vi "325-340 Read and Compressor auto control(SubVI) - v1.vi"(11 "Instrument":T3={"325 Resource "="GPIB0::24::INSTR", "Input (0:A) 325"=0, "Heater Output (1:1) 325"=1, "340 Resource"="GPIB0::14::INSTR", "Input (0:A) 340"=1, "Heater Output (1:1) 340"=1, "340 Status"=refnum, "Instrument Type"=enum."PPMS", "quantum design"=refnum, "semaphore 325"=refnum, "TCP master instance"=refnum, "M24C Resource"="GPIB0::24::INSTR", "4G supply"="GPIB0::24::INSTR", "Temp Status 24C"=refnum, "Temp"=refnum, "9T信号"=refnum, "limit"={"Field limit"=0.0, "Field rate limit"=0.0, "Temp limit"=0.0, "Temp low limit"=0.0, "Temp rate limit "=0.0}, "4g supply status"=refnum, "vi路径"="", "in-plane"="", "out-plane"="", "in-plane signal"=FALSE, "out-plane signal"=FALSE, "in plane 信号"=refnum, "pzt volt"=refnum, "Aborting"=refnum, "数据文件"=refnum, "warning"=refnum, "750 visa"="", "750 rotate"="", "335 Status 2"=refnum, "335 Resource "="GPIB0::24::INSTR", "Input (0:A) 335"=0, "Input (0:B) 335"=1, "Heater Output (1:1) 335"=1, "semaphore 340"=refnum, "semaphore 335"=refnum, "325 Status"=refnum} {"Heater Output (1:1) 335" items=["1"=1, "2"=2]; "Input (0:B) 335" items=["A", "B"]; "Input (0:A) 335" items=["A", "B"]; "Heater Output (1:1) 325" items=["1"=1, "2"=2]; "Input (0:A) 325" items=["A", "B"]; "Input (0:A) 340" items=["A", "B", "C", "D"]; "Heater Output (1:1) 340" items=["1", "2"]}) -> (3 "output cluster":T2 {"?" items=["Unknow", "Stable", "Following Warm", "Following Cold", "Unfollowing"]; "?" items=["Unknow", "Stable", "Following Warm", "Following Cold", "Unfollowing"]})   [LabVIEW 2019, in "Get value.lvlib"]
uses:
  Get value.lvlib
  ctl/Instrument.ctl
  <vilib>/NI/Modbus Library/API/Master/Modbus Master.lvclass
  ctl/335 state.ctl
  ctl/Instrument Type.ctl
  C:/Users/whmfc/Desktop/MEASURE/lib/QDInstrument.dll
  lib/QDInstrument.dll
  ctl/limit.ctl
  ctl/9T mag field stauts.ctl
  ctl/warning.ctl
  lib/Lake Shore 325/Lake Shore 325.lvlib
  lib/Lake Shore 340/Lake Shore Cryotronics 340.lvlib
panel:
  out "下拉列表 2":T1=2 items=["Unknow", "Stable", "Following Warm", "Following Cold", "Unfollowing"]
  out "下拉列表":T1=2 items=["Unknow", "Stable", "Following Warm", "Following Cold", "Unfollowing"]
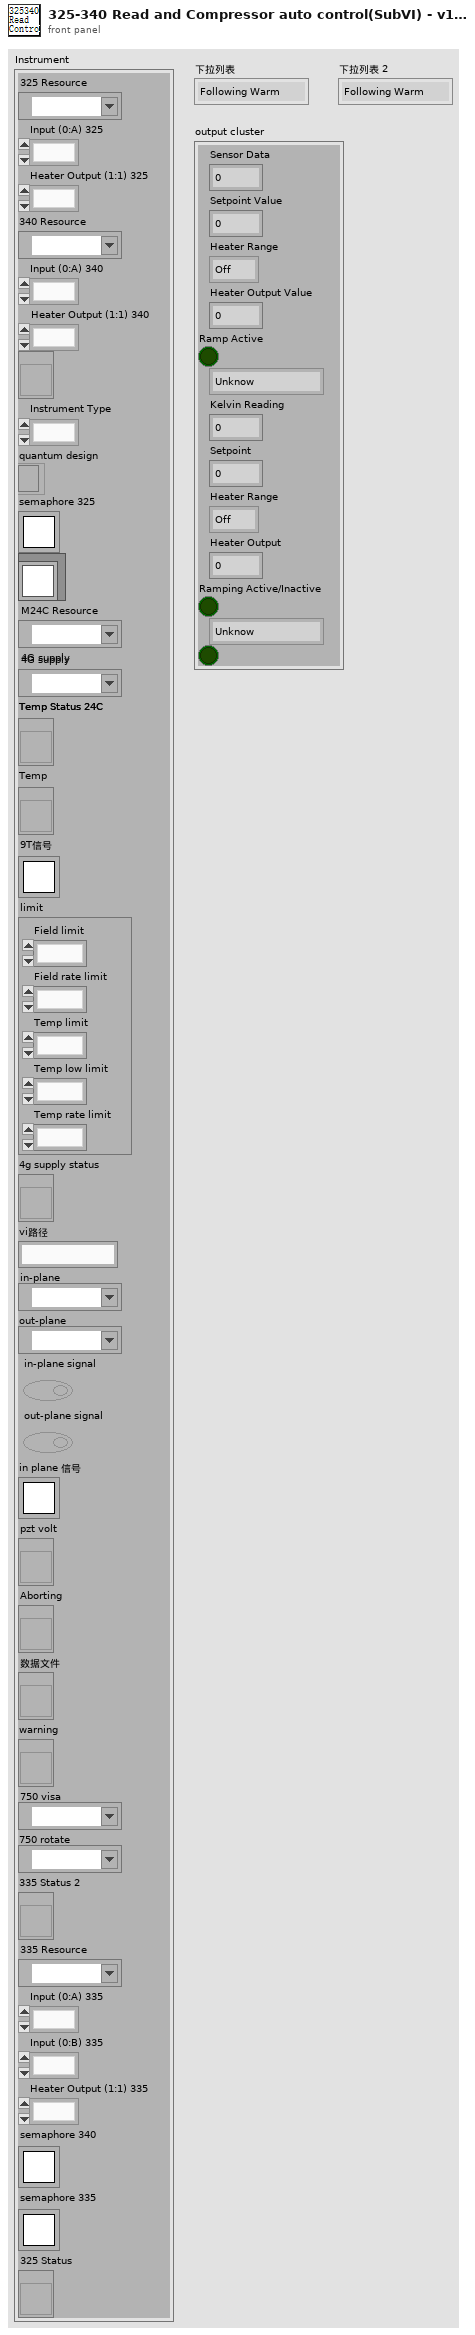
[diagram p1: front panel]
types:
  T1 = typedef "335 state.ctl" = u16
  T2 = cluster{"Sensor Data":dbl, "Setpoint Value":dbl, "Heater Range":enum16{"Off", "Low", "High"}, "Heater Output Value":dbl, "Ramp Active":bool, T1, "Kelvin Reading":dbl, "Setpoint":dbl, "Heater Range":enum16{"Off", "1", "2", "3", "4", "5"}, "Heater Output":dbl, "Ramping Active/Inactive":bool, T1, bool}
  T3 = typedef "Instrument.ctl" = cluster{"325 Resource ":refnum<visa-resource-name>, "Input (0:A) 325":u16, "Heater Output (1:1) 325":u16, "340 Resource":refnum<visa-resource-name>, "Input (0:A) 340":u16, "Heater Output (1:1) 340":u16, "340 Status":refnum<vi>, "Instrument Type":T4, "quantum design":refnum<k24>, "semaphore 325":T5, "TCP master instance":refnum<class "Modbus Master.lvclass">, "M24C Resource":refnum<visa-resource-name>, "4G supply":refnum<visa-resource-name>, "Temp Status 24C":refnum<vi>, "Temp":refnum<vi>, "9T信号":T5, "limit":T6, "4g supply status":refnum<vi>, "vi路径":string, "in-plane":refnum<visa-resource-name>, "out-plane":refnum<visa-resource-name>, "in-plane signal":bool, "out-plane signal":bool, "in plane 信号":T5, "pzt volt":refnum<vi>, "Aborting":refnum<vi>, "数据文件":refnum<vi>, "warning":refnum<vi>, "750 visa":refnum<visa-resource-name>, "750 rotate":refnum<visa-resource-name>, "335 Status 2":refnum<vi>, "335 Resource ":refnum<visa-resource-name>, "Input (0:A) 335":u16, "Input (0:B) 335":u16, "Heater Output (1:1) 335":u16, "semaphore 340":T5, "semaphore 335":T5, "325 Status":refnum<vi>}
  T4 = typedef "Instrument Type.ctl" = enum16{"PPMS", "VersaLab", "DynaCool", "SVSM", "PPMS-Rotate", "Lakeshore335", "lengtou2", "9T mag", "9T cmag rotate", "test"}
  T5 = typedef "Semaphore RefNum" = refnum<k1>
  T6 = typedef "limit.ctl" = cluster{"Field limit":dbl, "Field rate limit":dbl, "Temp limit":dbl, "Temp low limit":dbl, "Temp rate limit ":dbl}
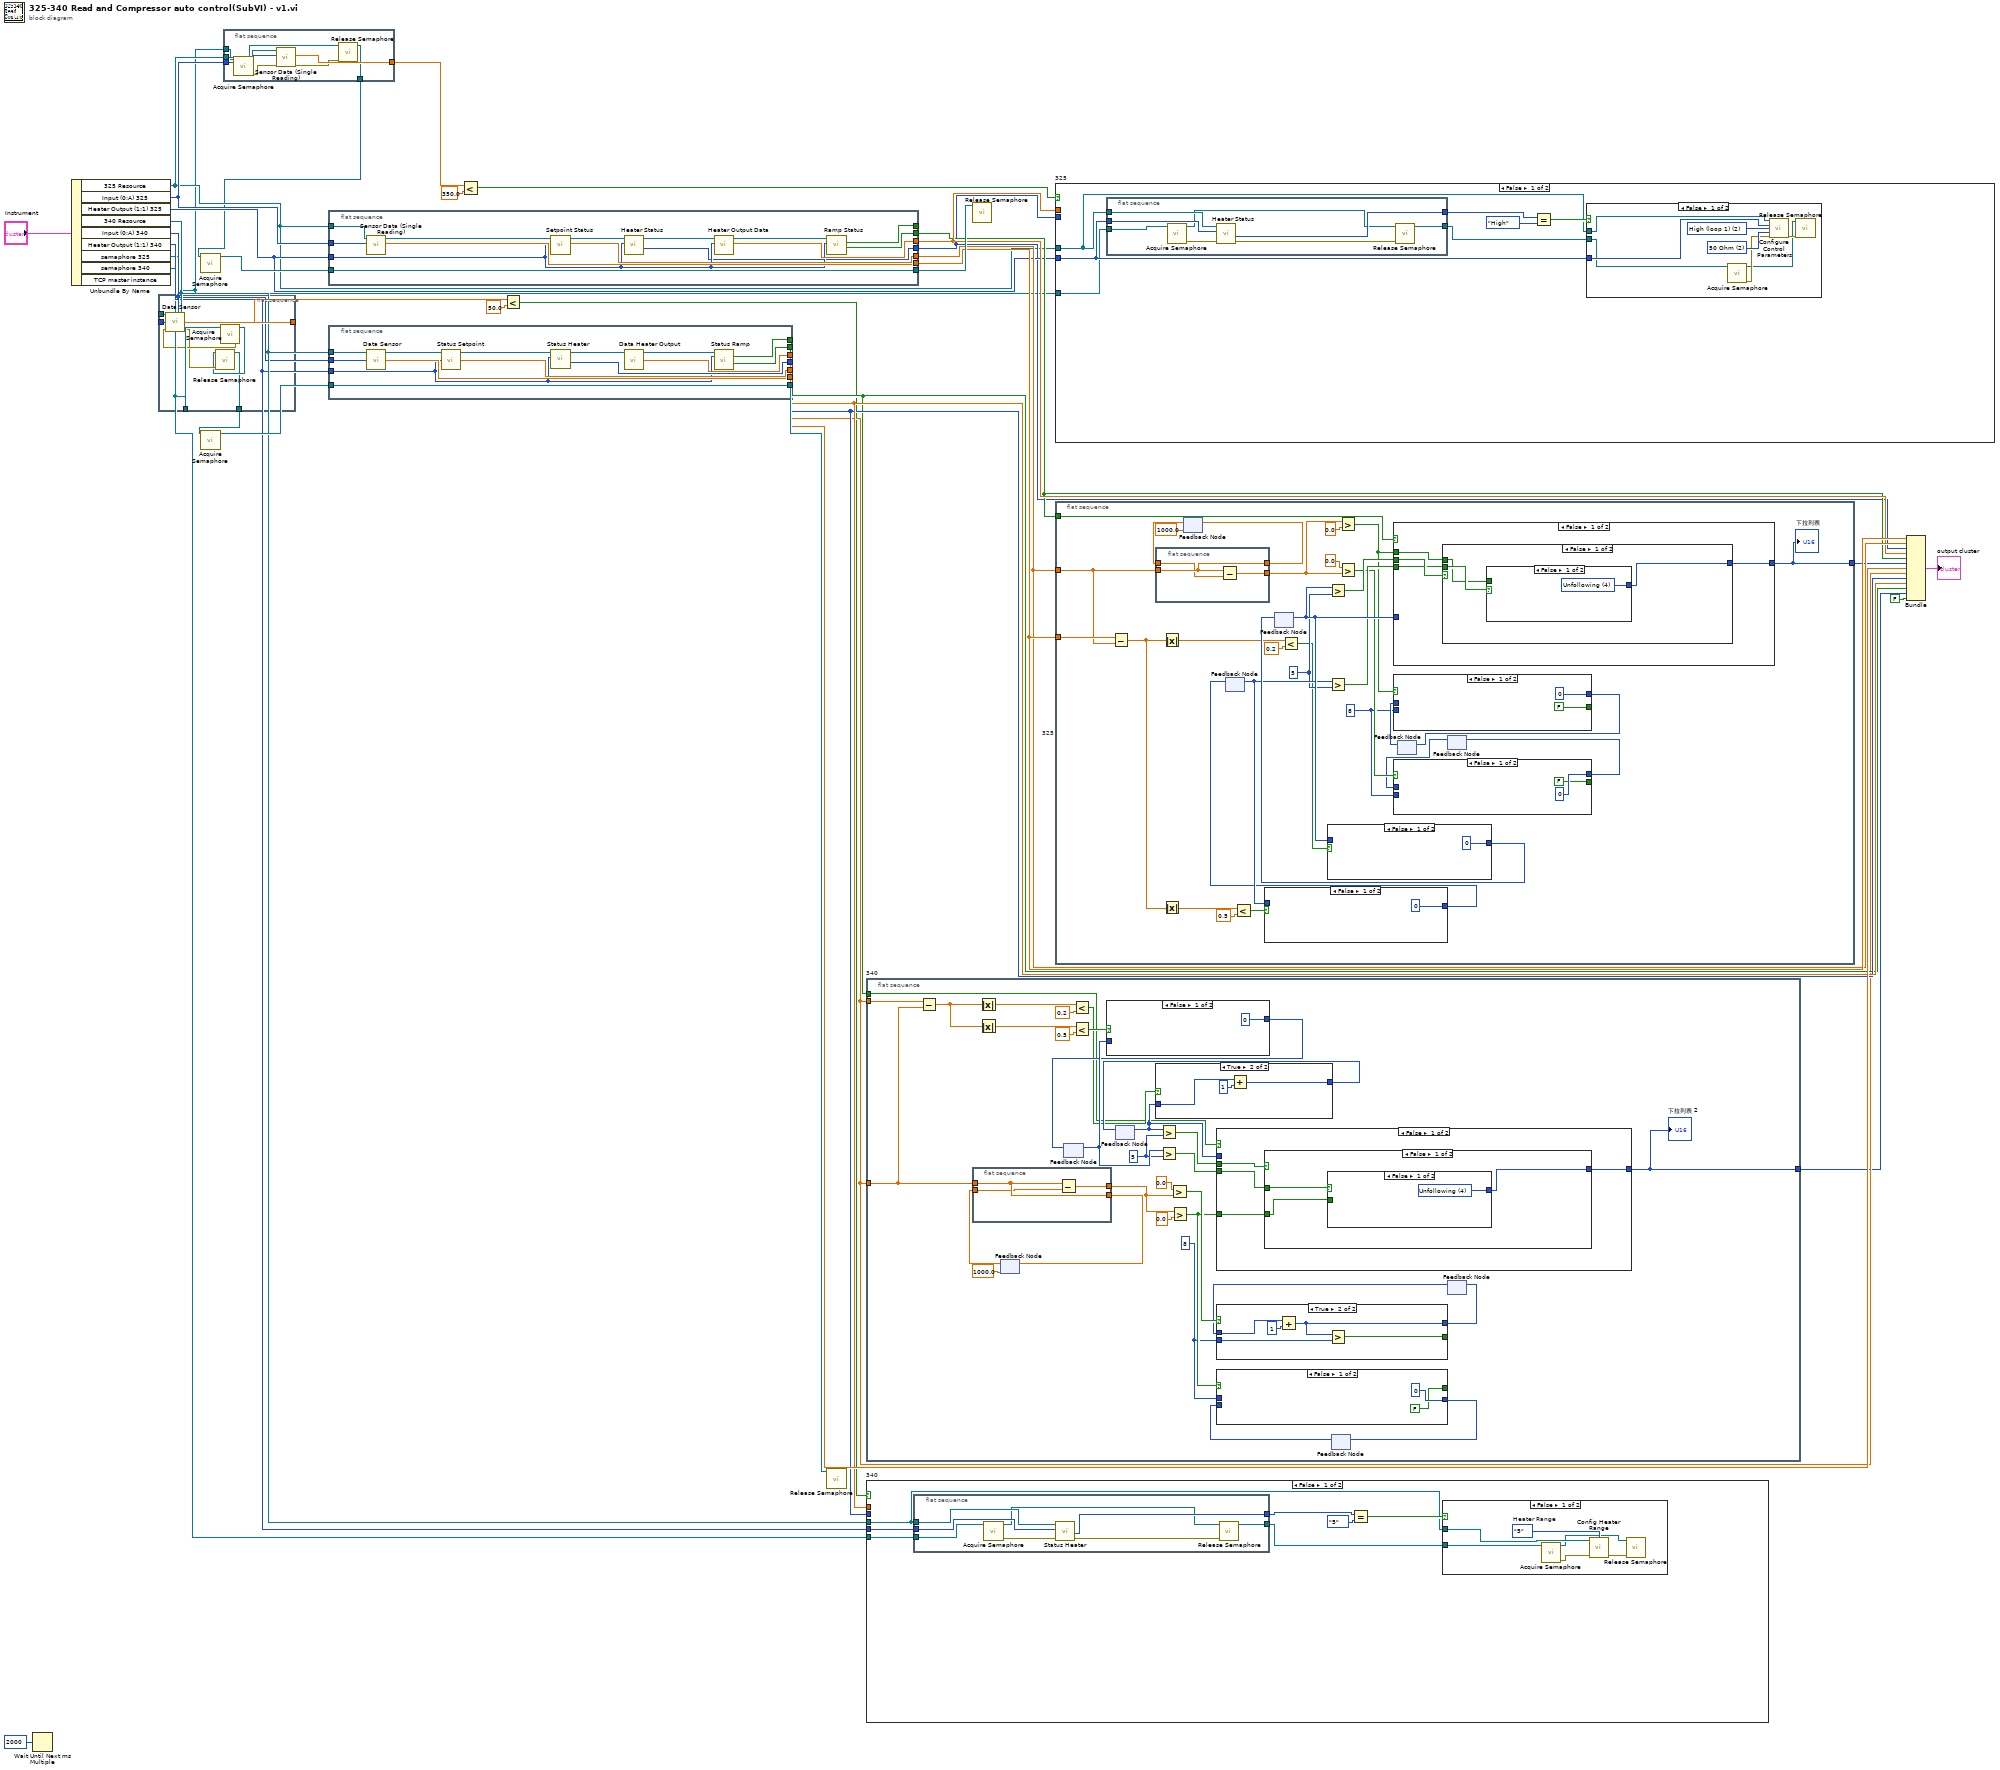
[diagram p0: block diagram]
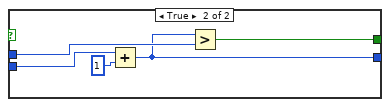
[diagram p2: hidden frame]
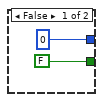
[diagram p3: hidden frame]
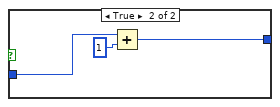
[diagram p4: hidden frame]
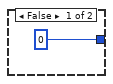
[diagram p5: hidden frame]
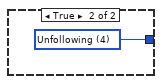
[diagram p6: hidden frame]
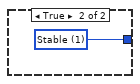
[diagram p7: hidden frame]
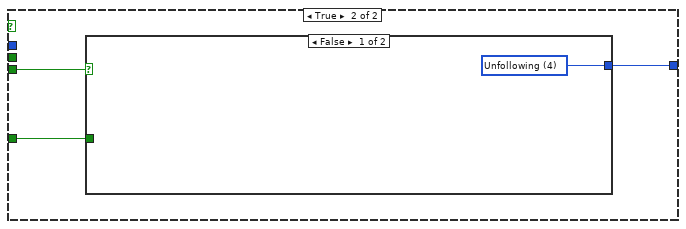
[diagram p8: hidden frame]
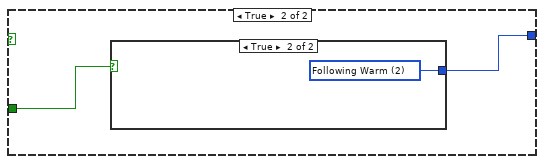
[diagram p9: hidden frame]
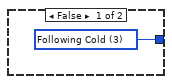
[diagram p10: hidden frame]
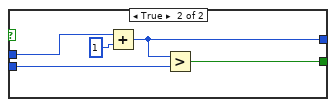
[diagram p11: hidden frame]
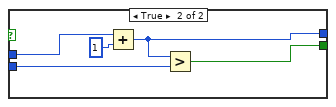
[diagram p12: hidden frame]
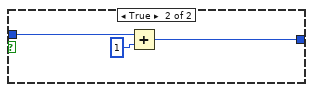
[diagram p13: hidden frame]
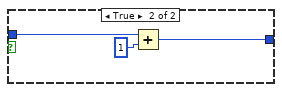
[diagram p14: hidden frame]
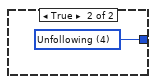
[diagram p15: hidden frame]
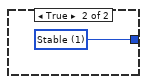
[diagram p16: hidden frame]
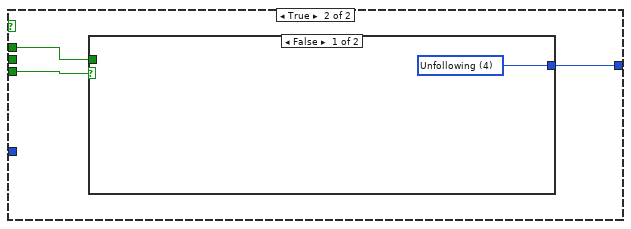
[diagram p17: hidden frame]
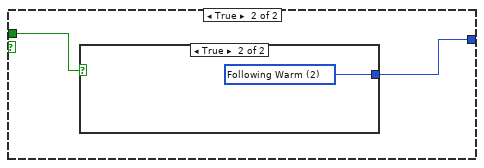
[diagram p18: hidden frame]
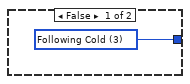
[diagram p19: hidden frame]
diagram:
  n1 = Wait Until Next ms Multiple(millisecond multiple=u32 2000) -> ()  [unwired: 1 out]
  n2 = Unbundle By Name("Instrument") -> ("325 Resource"=w5:refnum<visa-resource-name>, "Input (0:A) 325"=w7:u16, "Heater Output (1:1) 325"=w21:u16, "340 Resource"=w14:refnum<visa-resource-name>, "Input (0:A) 340"=w13:u16, "Heater Output (1:1) 340"=w10:u16, "semaphore 325"=w3:T5, "semaphore 340"=w2:T5)  [unwired: 1 out]
  n3 = flat-sequence {
    tunnel: [w44] -> w15
    tunnel: w14 -> [w43]
    tunnel: w13 -> [w42]
    tunnel: w2 -> [w41]
    tunnel: [w37] -> w1
    frame #0 {
      n4 = call <vilib>:"Acquire Semaphore.vi"("semaphore"=w41) -> ("error out"=w40:errorcluster, "semaphore out"=w38:T5)  [unwired: 4 in, 1 out]
      n5 = call "Data Sensor.vi"("VISA resource name"=w43, "Input (0: A)"=w42, "error in (no error)"=w40) -> ("Kelvin Reading"=w44:dbl, "error out"=w39:errorcluster)  [unwired: 8 in, 3 out]
      n6 = call <vilib>:"Release Semaphore.vi"("error in (no error)"=w39, "semaphore"=w38) -> ("semaphore out"=w37:T5)  [unwired: 4 in, 1 out]
    }
  }
  n7 = call <vilib>:"Acquire Semaphore.vi"("semaphore"=w4) -> ("semaphore out"=w35:T5)  [unwired: 4 in, 2 out]
  n8 = call <vilib>:"Acquire Semaphore.vi"("semaphore"=w1) -> ("semaphore out"=w32:T5)  [unwired: 4 in, 2 out]
  n9 = flat-sequence {
    tunnel: [w52] -> w8
    tunnel: w7 -> [w51]
    tunnel: w5 -> [w50]
    tunnel: [w46] -> w4
    tunnel: w3 -> [w45]
    frame #0 {
      n10 = call <vilib>:"Acquire Semaphore.vi"("semaphore"=w45) -> ("error out"=w49:errorcluster, "semaphore out"=w47:T5)  [unwired: 4 in, 1 out]
      n11 = call "Sensor Data (Single Reading).vi"("error in (no error)"=w49, "Sensor Input (0:A)"=w51, "VISA resource name"=w50) -> ("error out"=w48:errorcluster, "Sensor Data"=w52:dbl)  [unwired: 6 in, 1 out]
      n12 = call <vilib>:"Release Semaphore.vi"("error in (no error)"=w48, "semaphore"=w47) -> ("semaphore out"=w46:T5)  [unwired: 4 in, 1 out]
    }
  }
  n13 = flat-sequence {
    tunnel: [w56] -> w30
    tunnel: w35 -> [w66]
    tunnel: [w66] -> w36
    tunnel: w21 -> [w55]
    tunnel: w5 -> [w57]
    tunnel: w7 -> [w54]
    tunnel: [w61] -> w25
    tunnel: [w60] -> _
    tunnel: [w59] -> w29
    tunnel: [w53] -> w20
    tunnel: [w58] -> w28
    frame #0 {
      n14 = call "Sensor Data (Single Reading).vi"("Sensor Input (0:A)"=w54, "VISA resource name"=w57) -> ("Sensor Data"=w56:dbl, "VISA resource name out"=w64:refnum<visa-resource-name>)  [unwired: 7 in, 1 out]
      n15 = call "Setpoint Status.vi"("Loop (1:Loop 1)"=w55, "VISA resource name"=w64) -> ("Setpoint Value"=w59:dbl, "VISA resource name out"=w62:refnum<visa-resource-name>)  [unwired: 7 in, 1 out]
      n16 = call "Heater Status.vi"("Loop (1:Loop 1)"=w55, "VISA resource name"=w62) -> ("Heater Range"=w53:enum16{"Off", "Low", "High"}, "VISA resource name out"=w63:refnum<visa-resource-name>)  [unwired: 7 in, 1 out]
      n17 = call "Heater Output Data.vi"("Loop (1:Loop 1)"=w55, "VISA resource name"=w63) -> ("Heater Output Value"=w58:dbl, "VISA resource name out"=w65:refnum<visa-resource-name>)  [unwired: 7 in, 1 out]
      n18 = call "Ramp Status.vi"("Loop (1:Loop 1)"=w55, "VISA resource name"=w65) -> ("Ramp Active"=w61:bool, "Ramp On"=w60:bool)  [unwired: 5 in, 3 out]
    }
  }
  n19 = flat-sequence {
    tunnel: [w77] -> w17
    tunnel: w14 -> [w79]
    tunnel: w32 -> [w80]
    tunnel: [w80] -> w33
    tunnel: w13 -> [w68]
    tunnel: [w78] -> w18
    tunnel: [w76] -> w27
    tunnel: [w74] -> _
    tunnel: [w73] -> w26
    tunnel: w10 -> [w67]
    tunnel: [w69] -> w19
    frame #0 {
      n20 = call "Data Sensor.vi"("VISA resource name"=w79, "Input (0: A)"=w68) -> ("VISA resource name out"=w75:refnum<visa-resource-name>, "Kelvin Reading"=w76:dbl)  [unwired: 9 in, 3 out]
      n21 = call "Status Setpoint.vi"("VISA resource name"=w75, "Loop (0: 1)"=w67) -> ("VISA resource name out"=w71:refnum<visa-resource-name>, "Setpoint"=w77:dbl)  [unwired: 11 in, 1 out]
      n22 = call "Status Heater.vi"("Loop (1:Loop 1)"=w67, "VISA resource name"=w71) -> ("Heater Range"=w69:enum16{"Off", "1", "2", "3", "4", "5"}, "VISA resource name out"=w70:refnum<visa-resource-name>)  [unwired: 7 in, 1 out]
      n23 = call "Data Heater Output.vi"("VISA resource name"=w70) -> ("VISA resource name out"=w72:refnum<visa-resource-name>, "Heater Output"=w73:dbl)  [unwired: 12 in, 1 out]
      n24 = call "Status Ramp.vi"("VISA resource name"=w72, "Loop (0: 1)"=w67) -> ("Ramping On/Off"=w74:bool, "Ramping Active/Inactive"=w78:bool)  [unwired: 9 in, 3 out]
    }
  }
  n25 = Less?(x=w8, y=350.0) -> (x < y?=w6:bool)
  n26 = Less?(x=w15, y=50.0) -> (x < y?=w11:bool)
  n27 = call <vilib>:"Release Semaphore.vi"("semaphore"=w33) -> ()  [unwired: 5 in, 2 out]
  n28 = flat-sequence "340" {
    tunnel: w17 -> [w84]
    tunnel: w17 -> [w83]
    tunnel: w18 -> [w82]
    tunnel: [w81] -> w16
    frame #0 {
      w85 = 8 ("y")
      w99 = 5 ("y")
      n29 = Subtract(x=w84, y=w83) -> (x-y=w97:dbl)
      n30 = flat-sequence {
        tunnel: w83 -> [w128]
        tunnel: [w128] -> w106
        tunnel: w107 -> [w127]
        tunnel: [w126] -> w111
        frame #0 {
          n31 = Subtract(x=w128, y=w127) -> (x-y=w126:dbl)
        }
      }
      n32 = Absolute Value(x=w97) -> (abs(x)=w94:dbl)
      n33 = Absolute Value(x=w97) -> (abs(x)=w95:dbl)
      n34 = feedback #1(1000.0 ("Setpoint")) -> (w107:dbl)
      n35 = feedback-in #1(w106) -> ()
      n36 = feedback #2() -> (w103:i32)  [unwired: 1 in]
      n37 = Less?(x=w94, y=0.2) -> (x < y?=w93:bool)
      n38 = Less?(x=w95, y=0.5) -> (x < y?=w98:bool)
      n39 = case shown="False" w98 {
        tunnel: w103 -> [_ w132]
        tunnel: [0 w130] -> w102
        frame False {
        }
        frame True {
          n40 = Add(x=w132, y=1) -> (x+y=w130:i32)
        }
      }
      n41 = feedback-in #2(w102) -> ()
      n42 = feedback #3() -> (w105:i32)  [unwired: 1 in]
      n43 = case shown="True" w93 {
        tunnel: w105 -> [_ w136]
        tunnel: [0 w134] -> w104
        frame False {
        }
        frame True {
          n44 = Add(x=w136, y=1) -> (x+y=w134:i32)
        }
      }
      n45 = feedback-in #3(w104) -> ()
      n46 = Greater?(x=w105, y=w99) -> (0:w100:bool)
      n47 = Greater?(x=w103, y=w99) -> (0:w101:bool)
      n48 = Greater?(x=0.0, y=w111) -> (0:w91:bool)
      n49 = Greater?(x=w111, y=0.0) -> (0:w86:bool)
      n50 = case shown="False" w82 {
        tunnel: w105 -> [_ _]
        tunnel: w100 -> [w140 _]
        tunnel: w101 -> [w139 w149]
        tunnel: [w138 w148] -> w81
        tunnel: w86 -> [w137 w147]
        frame False {
          n51 = case shown="False" w140 {
            tunnel: [w142 w146] -> w138
            tunnel: w139 -> [w143 _]
            tunnel: w137 -> [w141 _]
            frame False {
              n52 = case shown="False" w143 {
                tunnel: [w144 w145] -> w142
                tunnel: w141 -> [_ _]
                frame False {
                  w144 = T1 4 items=["Unknow", "Stable", "Following Warm", "Following Cold", "Unfollowing"]
                }
                frame True {
                  w145 = T1 4 items=["Unknow", "Stable", "Following Warm", "Following Cold", "Unfollowing"]
                }
              }
            }
            frame True {
              w146 = T1 1 items=["Unknow", "Stable", "Following Warm", "Following Cold", "Unfollowing"]
            }
          }
        }
        frame True {
          n53 = case shown="False" w149 {
            tunnel: [w150 w151] -> w148
            tunnel: w147 -> [_ w152]
            frame False {
              w150 = T1 4 items=["Unknow", "Stable", "Following Warm", "Following Cold", "Unfollowing"]
            }
            frame True {
              n54 = case shown="True" w152 {
                tunnel: [w153 w154] -> w151
                frame False {
                  w153 = T1 3 items=["Unknow", "Stable", "Following Warm", "Following Cold", "Unfollowing"]
                }
                frame True {
                  w154 = T1 2 items=["Unknow", "Stable", "Following Warm", "Following Cold", "Unfollowing"]
                }
              }
            }
          }
        }
      }
      "下拉列表 2" <- w81
      n55 = feedback #4() -> (w88:i32)  [unwired: 1 in]
      n56 = case shown="False" w86 {
        tunnel: [0 w115] -> w87
        tunnel: w88 -> [_ w117]
        tunnel: w85 -> [_ w116]
        tunnel: [FALSE w114] -> _
        frame False {
        }
        frame True {
          n57 = Add(x=w117, y=1) -> (x+y=w115:i32)
          n58 = Greater?(x=w115, y=w116) -> (0:w114:bool)
        }
      }
      n59 = feedback-in #4(w87) -> ()
      n60 = feedback #5() -> (w89:i32)  [unwired: 1 in]
      n61 = case shown="True" w91 {
        tunnel: [0 w123] -> w90
        tunnel: w89 -> [_ w124]
        tunnel: w85 -> [_ w122]
        tunnel: [FALSE w121] -> _
        frame False {
        }
        frame True {
          n62 = Add(x=w124, y=1) -> (x+y=w123:i32)
          n63 = Greater?(x=w123, y=w122) -> (0:w121:bool)
        }
      }
      n64 = feedback-in #5(w90) -> ()
    }
  }
  n65 = case "340" shown="False" w11 {
    tunnel: w26 -> [_ w187]
    tunnel: w14 -> [w157 w184]
    tunnel: w2 -> [w155 w183]
    tunnel: w19 -> [_ w176]
    tunnel: w10 -> [w161 _]
    frame False {
      n66 = flat-sequence {
        tunnel: w161 -> [w169]
        tunnel: [w168] -> w160
        tunnel: w157 -> [w167]
        tunnel: w155 -> [w163]
        tunnel: [w162] -> w156
        frame #0 {
          n67 = call <vilib>:"Acquire Semaphore.vi"("semaphore"=w163) -> ("error out"=w165:errorcluster, "semaphore out"=w164:T5)  [unwired: 4 in, 1 out]
          n68 = call "Status Heater.vi"("error in (no error)"=w165, "Loop (1:Loop 1)"=w169, "VISA resource name"=w167) -> ("error out"=w166:errorcluster, "Heater Range"=w168:enum16{"Off", "1", "2", "3", "4", "5"})  [unwired: 6 in, 1 out]
          n69 = call <vilib>:"Release Semaphore.vi"("error in (no error)"=w166, "semaphore"=w164) -> ("semaphore out"=w162:T5)  [unwired: 4 in, 1 out]
        }
      }
      n70 = Equal?(x=w160, y=enum16{"Off", "1", "2", "3", "4", "5"}."5" ("Heater Range")) -> (x = y?=w158:bool)
      n71 = case shown="False" w158 {
        tunnel: w157 -> [w174 _]
        tunnel: w156 -> [w172 _]
        frame False {
          w175 = enum16{"Off", "1", "2", "3", "4", "5"}."5"  # Heater Range
          n72 = call <vilib>:"Acquire Semaphore.vi"("semaphore"=w172) -> ("error out"=w171:errorcluster, "semaphore out"=w170:T5)  [unwired: 4 in, 1 out]
          n73 = call "Config Heater Range.vi"("VISA resource name"=w174, "Heater Range (0: Off)"=w175, "error in (no error)"=w171) -> ("error out"=w173:errorcluster)  [unwired: 11 in, 1 out]
          n74 = call <vilib>:"Release Semaphore.vi"("error in (no error)"=w173, "semaphore"=w170) -> ()  [unwired: 4 in, 2 out]
        }
        frame True {
        }
      }
    }
    frame True {
      n75 = Less?(x=w187, y=5.0) -> (x < y?=w178:bool)
      n76 = Greater?(x=w187, y=80.0) -> (0:w185:bool)
      n77 = feedback #6(0) -> (w179:i32)
      n78 = Greater?(x=w179, y=3) -> (0:w181:bool)
      n79 = case shown="True" w181 {
        tunnel: w185 -> [_ w198]
        tunnel: w184 -> [_ w197]
        tunnel: w183 -> [_ w196]
        tunnel: [w189 w195] -> w180
        tunnel: w179 -> [w191 w194]
        tunnel: w178 -> [_ w193]
        tunnel: w176 -> [_ w192]
        frame False {
          n80 = Add(x=1, y=w191) -> (x+y=w189:i32)
        }
        frame True {
          n81 = case shown="True" w198 {
            tunnel: w197 -> [w204 w255]
            tunnel: w196 -> [w201 w254]
            tunnel: [w203 w253] -> w195
            tunnel: w194 -> [w202 w252]
            tunnel: w193 -> [w200 _]
            tunnel: w192 -> [w199 w251]
            frame False {
              n82 = case shown="True" w200 {
                tunnel: w204 -> [_ w211]
                tunnel: [w205 w212] -> w203
                tunnel: w202 -> [w207 w209]
                tunnel: w201 -> [_ w210]
                tunnel: w199 -> [_ w208]
                frame False {
                  n83 = Add(x=1, y=w207) -> (x+y=w205:i32)
                }
                frame True {
                  n84 = case shown="\"5\"" w208 {
                    tunnel: w211 -> [w214 _ w224 w232 w239 w245]
                    tunnel: w210 -> [w213 _ w223 w231 w238 w247]
                    tunnel: [0 w220 0 0 0 0] -> w212
                    tunnel: w209 -> [_ w221 _ _ _ _]
                    frame "Off" {
                      w216 = enum16{"Off", "1", "2", "3", "4", "5"}."1"  # Heater Range
                      n85 = call <vilib>:"Acquire Semaphore.vi"("semaphore"=w213) -> ("error out"=w219:errorcluster, "semaphore out"=w217:T5)  [unwired: 4 in, 1 out]
                      n86 = call "Config Heater Range.vi"("VISA resource name"=w214, "Heater Range (0: Off)"=w216, "error in (no error)"=w219) -> ("error out"=w218:errorcluster)  [unwired: 11 in, 1 out]
                      n87 = call <vilib>:"Release Semaphore.vi"("error in (no error)"=w218, "semaphore"=w217) -> ()  [unwired: 4 in, 2 out]
                    }
                    frame "1", Default {
                      n88 = Add(x=1, y=w221) -> (x+y=w220:i32)
                    }
                    frame "2" {
                      w225 = enum16{"Off", "1", "2", "3", "4", "5"}."1"  # Heater Range
                      n89 = call <vilib>:"Acquire Semaphore.vi"("semaphore"=w223) -> ("error out"=w228:errorcluster, "semaphore out"=w226:T5)  [unwired: 4 in, 1 out]
                      n90 = call "Config Heater Range.vi"("VISA resource name"=w224, "Heater Range (0: Off)"=w225, "error in (no error)"=w228) -> ("error out"=w227:errorcluster)  [unwired: 11 in, 1 out]
                      n91 = call <vilib>:"Release Semaphore.vi"("error in (no error)"=w227, "semaphore"=w226) -> ()  [unwired: 4 in, 2 out]
                    }
                    frame "3" {
                      w233 = enum16{"Off", "1", "2", "3", "4", "5"}."2"  # Heater Range
                      n92 = call <vilib>:"Acquire Semaphore.vi"("semaphore"=w231) -> ("error out"=w236:errorcluster, "semaphore out"=w234:T5)  [unwired: 4 in, 1 out]
                      n93 = call "Config Heater Range.vi"("VISA resource name"=w232, "Heater Range (0: Off)"=w233, "error in (no error)"=w236) -> ("error out"=w235:errorcluster)  [unwired: 11 in, 1 out]
                      n94 = call <vilib>:"Release Semaphore.vi"("error in (no error)"=w235, "semaphore"=w234) -> ()  [unwired: 4 in, 2 out]
                    }
                    frame "4" {
                      w240 = enum16{"Off", "1", "2", "3", "4", "5"}."3"  # Heater Range
                      n95 = call <vilib>:"Acquire Semaphore.vi"("semaphore"=w238) -> ("error out"=w243:errorcluster, "semaphore out"=w241:T5)  [unwired: 4 in, 1 out]
                      n96 = call "Config Heater Range.vi"("VISA resource name"=w239, "Heater Range (0: Off)"=w240, "error in (no error)"=w243) -> ("error out"=w242:errorcluster)  [unwired: 11 in, 1 out]
                      n97 = call <vilib>:"Release Semaphore.vi"("error in (no error)"=w242, "semaphore"=w241) -> ()  [unwired: 4 in, 2 out]
                    }
                    frame "5" {
                      w246 = enum16{"Off", "1", "2", "3", "4", "5"}."4"  # Heater Range
                      n98 = call <vilib>:"Acquire Semaphore.vi"("semaphore"=w247) -> ("error out"=w250:errorcluster, "semaphore out"=w248:T5)  [unwired: 4 in, 1 out]
                      n99 = call "Config Heater Range.vi"("VISA resource name"=w245, "Heater Range (0: Off)"=w246, "error in (no error)"=w250) -> ("error out"=w249:errorcluster)  [unwired: 11 in, 1 out]
                      n100 = call <vilib>:"Release Semaphore.vi"("error in (no error)"=w249, "semaphore"=w248) -> ()  [unwired: 4 in, 2 out]
                    }
                  }
                }
              }
            }
            frame True {
              n101 = case shown="\"4\"" w251 {
                tunnel: w255 -> [w257 w264 w271 w279 w286 _]
                tunnel: w254 -> [w256 w266 w270 w278 w285 _]
                tunnel: [0 0 0 0 0 w291] -> w253
                tunnel: w252 -> [_ _ _ _ _ w292]
                frame "Off" {
                  w259 = enum16{"Off", "1", "2", "3", "4", "5"}."1"  # Heater Range
                  n102 = call <vilib>:"Acquire Semaphore.vi"("semaphore"=w256) -> ("error out"=w262:errorcluster, "semaphore out"=w260:T5)  [unwired: 4 in, 1 out]
                  n103 = call "Config Heater Range.vi"("VISA resource name"=w257, "Heater Range (0: Off)"=w259, "error in (no error)"=w262) -> ("error out"=w261:errorcluster)  [unwired: 11 in, 1 out]
                  n104 = call <vilib>:"Release Semaphore.vi"("error in (no error)"=w261, "semaphore"=w260) -> ()  [unwired: 4 in, 2 out]
                }
                frame "1", Default {
                  w265 = enum16{"Off", "1", "2", "3", "4", "5"}."2"  # Heater Range
                  n105 = call <vilib>:"Acquire Semaphore.vi"("semaphore"=w266) -> ("error out"=w269:errorcluster, "semaphore out"=w267:T5)  [unwired: 4 in, 1 out]
                  n106 = call "Config Heater Range.vi"("VISA resource name"=w264, "Heater Range (0: Off)"=w265, "error in (no error)"=w269) -> ("error out"=w268:errorcluster)  [unwired: 11 in, 1 out]
                  n107 = call <vilib>:"Release Semaphore.vi"("error in (no error)"=w268, "semaphore"=w267) -> ()  [unwired: 4 in, 2 out]
                }
                frame "2" {
                  w272 = enum16{"Off", "1", "2", "3", "4", "5"}."3"  # Heater Range
                  n108 = call <vilib>:"Acquire Semaphore.vi"("semaphore"=w270) -> ("error out"=w275:errorcluster, "semaphore out"=w273:T5)  [unwired: 4 in, 1 out]
                  n109 = call "Config Heater Range.vi"("VISA resource name"=w271, "Heater Range (0: Off)"=w272, "error in (no error)"=w275) -> ("error out"=w274:errorcluster)  [unwired: 11 in, 1 out]
                  n110 = call <vilib>:"Release Semaphore.vi"("error in (no error)"=w274, "semaphore"=w273) -> ()  [unwired: 4 in, 2 out]
                }
                frame "3" {
                  w280 = enum16{"Off", "1", "2", "3", "4", "5"}."4"  # Heater Range
                  n111 = call <vilib>:"Acquire Semaphore.vi"("semaphore"=w278) -> ("error out"=w283:errorcluster, "semaphore out"=w281:T5)  [unwired: 4 in, 1 out]
                  n112 = call "Config Heater Range.vi"("VISA resource name"=w279, "Heater Range (0: Off)"=w280, "error in (no error)"=w283) -> ("error out"=w282:errorcluster)  [unwired: 11 in, 1 out]
                  n113 = call <vilib>:"Release Semaphore.vi"("error in (no error)"=w282, "semaphore"=w281) -> ()  [unwired: 4 in, 2 out]
                }
                frame "4" {
                  w287 = enum16{"Off", "1", "2", "3", "4", "5"}."5"  # Heater Range
                  n114 = call <vilib>:"Acquire Semaphore.vi"("semaphore"=w285) -> ("error out"=w290:errorcluster, "semaphore out"=w288:T5)  [unwired: 4 in, 1 out]
                  n115 = call "Config Heater Range.vi"("VISA resource name"=w286, "Heater Range (0: Off)"=w287, "error in (no error)"=w290) -> ("error out"=w289:errorcluster)  [unwired: 11 in, 1 out]
                  n116 = call <vilib>:"Release Semaphore.vi"("error in (no error)"=w289, "semaphore"=w288) -> ()  [unwired: 4 in, 2 out]
                }
                frame "5" {
                  n117 = Add(x=1, y=w292) -> (x+y=w291:i32)
                }
              }
            }
          }
        }
      }
      n118 = feedback-in #6(w180) -> ()
    }
  }
  n119 = call <vilib>:"Release Semaphore.vi"("semaphore"=w36) -> ()  [unwired: 5 in, 2 out]
  n120 = case "325" shown="False" w6 {
    tunnel: w28 -> [_ w329]
    tunnel: w20 -> [_ w326]
    tunnel: w5 -> [w297 w325]
    tunnel: w21 -> [w296 w324]
    tunnel: w3 -> [w294 w317]
    frame False {
      n121 = flat-sequence {
        tunnel: [w308] -> w299
        tunnel: w297 -> [w307]
        tunnel: w296 -> [w306]
        tunnel: w294 -> [w304]
        tunnel: [w301] -> w295
        frame #0 {
          n122 = call <vilib>:"Acquire Semaphore.vi"("semaphore"=w304) -> ("error out"=w305:errorcluster, "semaphore out"=w302:T5)  [unwired: 4 in, 1 out]
          n123 = call "Heater Status.vi"("error in (no error)"=w305, "Loop (1:Loop 1)"=w306, "VISA resource name"=w307) -> ("error out"=w303:errorcluster, "Heater Range"=w308:enum16{"Off", "Low", "High"})  [unwired: 6 in, 1 out]
          n124 = call <vilib>:"Release Semaphore.vi"("error in (no error)"=w303, "semaphore"=w302) -> ("semaphore out"=w301:T5)  [unwired: 4 in, 1 out]
        }
      }
      n125 = Equal?(x=w299, y=enum16{"Off", "Low", "High"}."High" ("Heater Range")) -> (x = y?=w300:bool)
      n126 = case shown="False" w300 {
        tunnel: w297 -> [w315 _]
        tunnel: w296 -> [w313 _]
        tunnel: w295 -> [w312 _]
        frame False {
          w314 = u16 2 items=["Off", "Low (loop 1) or On (loop 2)", "High (loop 1)"] ("Heater Range (0:Off)")
          w316 = u16 2 items=["25 Ohm"=1, "50 Ohm"=2] ("Heater Resistance (1:25 Ohm)")
          n127 = call <vilib>:"Acquire Semaphore.vi"("semaphore"=w312) -> ("error out"=w311:errorcluster, "semaphore out"=w309:T5)  [unwired: 4 in, 1 out]
          n128 = call "Configure Control Parameters.vi"("VISA resource name"=w315, "Loop (1:Loop 1)"=w313, "Heater Range (0:Off)"=w314, "Heater Resistance (1:25 Ohm)"=w316, "error in (no error)"=w311) -> ("error out"=w310:errorcluster)  [unwired: 9 in, 1 out]
          n129 = call <vilib>:"Release Semaphore.vi"("error in (no error)"=w310, "semaphore"=w309) -> ()  [unwired: 4 in, 2 out]
        }
        frame True {
        }
      }
    }
    frame True {
      n130 = Less?(x=w329, y=5.0) -> (x < y?=w319:bool)
      n131 = Greater?(x=w329, y=80.0) -> (0:w327:bool)
      n132 = feedback #7(0) -> (w320:i32)
      n133 = Greater?(x=w320, y=3) -> (0:w322:bool)
      n134 = case shown="True" w322 {
        tunnel: w327 -> [_ w341]
        tunnel: w326 -> [_ w340]
        tunnel: w325 -> [_ w339]
        tunnel: w324 -> [_ w338]
        tunnel: w317 -> [_ w337]
        tunnel: [w331 w336] -> w321
        tunnel: w320 -> [w333 w335]
        tunnel: w319 -> [_ w334]
        frame False {
          n135 = Add(x=1, y=w333) -> (x+y=w331:i32)
        }
        frame True {
          n136 = case shown="True" w341 {
            tunnel: w340 -> [w348 w384]
            tunnel: w339 -> [w347 w383]
            tunnel: w338 -> [w346 w382]
            tunnel: w337 -> [w343 w381]
            tunnel: [w345 w380] -> w336
            tunnel: w335 -> [w344 w379]
            tunnel: w334 -> [w342 _]
            frame False {
              n137 = case shown="True" w342 {
                tunnel: w348 -> [_ w352]
                tunnel: w347 -> [_ w357]
                tunnel: w346 -> [_ w356]
                tunnel: [w349 w355] -> w345
                tunnel: w344 -> [w351 w354]
                tunnel: w343 -> [_ w353]
                frame False {
                  n138 = Add(x=1, y=w351) -> (x+y=w349:i32)
                }
                frame True {
                  n139 = case shown="\"Off\"" w352 {
                    tunnel: w357 -> [w363 _ w375]
                    tunnel: w356 -> [w360 _ w372]
                    tunnel: [0 w367 0] -> w355
                    tunnel: w354 -> [_ w369 _]
                    tunnel: w353 -> [w362 _ w373]
                    frame "Off" {
                      w358 = u16 1 items=["Off", "Low (loop 1) or On (loop 2)", "High (loop 1)"] ("Heater Range (0:Off)")
                      w364 = u16 2 items=["25 Ohm"=1, "50 Ohm"=2] ("Heater Resistance (1:25 Ohm)")
                      n140 = call <vilib>:"Acquire Semaphore.vi"("semaphore"=w362) -> ("error out"=w366:errorcluster, "semaphore out"=w361:T5)  [unwired: 4 in, 1 out]
                      n141 = call "Configure Control Parameters.vi"("VISA resource name"=w363, "Loop (1:Loop 1)"=w360, "Heater Range (0:Off)"=w358, "Heater Resistance (1:25 Ohm)"=w364, "error in (no error)"=w366) -> ("error out"=w365:errorcluster)  [unwired: 9 in, 1 out]
                      n142 = call <vilib>:"Release Semaphore.vi"("error in (no error)"=w365, "semaphore"=w361) -> ()  [unwired: 4 in, 2 out]
                    }
                    frame "Low", Default {
                      n143 = Add(x=1, y=w369) -> (x+y=w367:i32)
                    }
                    frame "High" {
                      w370 = u16 1 items=["Off", "Low (loop 1) or On (loop 2)", "High (loop 1)"] ("Heater Range (0:Off)")
                      w371 = u16 2 items=["25 Ohm"=1, "50 Ohm"=2] ("Heater Resistance (1:25 Ohm)")
                      n144 = call <vilib>:"Acquire Semaphore.vi"("semaphore"=w373) -> ("error out"=w378:errorcluster, "semaphore out"=w376:T5)  [unwired: 4 in, 1 out]
                      n145 = call "Configure Control Parameters.vi"("VISA resource name"=w375, "Loop (1:Loop 1)"=w372, "Heater Range (0:Off)"=w370, "Heater Resistance (1:25 Ohm)"=w371, "error in (no error)"=w378) -> ("error out"=w377:errorcluster)  [unwired: 9 in, 1 out]
                      n146 = call <vilib>:"Release Semaphore.vi"("error in (no error)"=w377, "semaphore"=w376) -> ()  [unwired: 4 in, 2 out]
                    }
                  }
                }
              }
            }
            frame True {
              n147 = case shown="\"Low\", Default" w384 {
                tunnel: w383 -> [w389 w402 _]
                tunnel: w382 -> [w388 w401 _]
                tunnel: w381 -> [w387 w397 _]
                tunnel: [0 0 w403] -> w380
                tunnel: w379 -> [_ _ w405]
                frame "Off" {
                  w385 = u16 1 items=["Off", "Low (loop 1) or On (loop 2)", "High (loop 1)"] ("Heater Range (0:Off)")
                  w390 = u16 2 items=["25 Ohm"=1, "50 Ohm"=2] ("Heater Resistance (1:25 Ohm)")
                  n148 = call <vilib>:"Acquire Semaphore.vi"("semaphore"=w387) -> ("error out"=w393:errorcluster, "semaphore out"=w391:T5)  [unwired: 4 in, 1 out]
                  n149 = call "Configure Control Parameters.vi"("VISA resource name"=w389, "Loop (1:Loop 1)"=w388, "Heater Range (0:Off)"=w385, "Heater Resistance (1:25 Ohm)"=w390, "error in (no error)"=w393) -> ("error out"=w392:errorcluster)  [unwired: 9 in, 1 out]
                  n150 = call <vilib>:"Release Semaphore.vi"("error in (no error)"=w392, "semaphore"=w391) -> ()  [unwired: 4 in, 2 out]
                }
                frame "Low", Default {
                  w394 = u16 2 items=["Off", "Low (loop 1) or On (loop 2)", "High (loop 1)"] ("Heater Range (0:Off)")
                  w395 = u16 2 items=["25 Ohm"=1, "50 Ohm"=2] ("Heater Resistance (1:25 Ohm)")
                  n151 = call <vilib>:"Acquire Semaphore.vi"("semaphore"=w397) -> ("error out"=w400:errorcluster, "semaphore out"=w398:T5)  [unwired: 4 in, 1 out]
                  n152 = call "Configure Control Parameters.vi"("VISA resource name"=w402, "Loop (1:Loop 1)"=w401, "Heater Range (0:Off)"=w394, "Heater Resistance (1:25 Ohm)"=w395, "error in (no error)"=w400) -> ("error out"=w399:errorcluster)  [unwired: 9 in, 1 out]
                  n153 = call <vilib>:"Release Semaphore.vi"("error in (no error)"=w399, "semaphore"=w398) -> ()  [unwired: 4 in, 2 out]
                }
                frame "High" {
                  n154 = Add(x=w405, y=1) -> (x+y=w403:i32)
                }
              }
            }
          }
        }
      }
      n155 = feedback-in #7(w321) -> ()
    }
  }
  n156 = flat-sequence "325" {
    tunnel: w30 -> [w409]
    tunnel: w29 -> [w408]
    tunnel: w25 -> [w407]
    tunnel: [w406] -> w23
    frame #0 {
      w410 = 8 ("y")
      w424 = 5 ("y")
      n157 = Subtract(x=w409, y=w408) -> (x-y=w422:dbl)
      n158 = flat-sequence {
        tunnel: w408 -> [w453]
        tunnel: [w453] -> w431
        tunnel: w432 -> [w452]
        tunnel: [w451] -> w436
        frame #0 {
          n159 = Subtract(x=w453, y=w452) -> (x-y=w451:dbl)
        }
      }
      n160 = Absolute Value(x=w422) -> (abs(x)=w419:dbl)
      n161 = Absolute Value(x=w422) -> (abs(x)=w420:dbl)
      n162 = feedback #8(1000.0 ("Setpoint")) -> (w432:dbl)
      n163 = feedback-in #8(w431) -> ()
      n164 = feedback #9() -> (w428:i32)  [unwired: 1 in]
      n165 = Less?(x=w420, y=0.5) -> (x < y?=w423:bool)
      n166 = case shown="False" w423 {
        tunnel: w428 -> [_ w457]
        tunnel: [0 w455] -> w427
        frame False {
        }
        frame True {
          n167 = Add(x=w457, y=1) -> (x+y=w455:i32)
        }
      }
      n168 = feedback-in #9(w427) -> ()
      n169 = feedback #10() -> (w430:i32)  [unwired: 1 in]
      n170 = Less?(x=w419, y=0.2) -> (x < y?=w418:bool)
      n171 = case shown="False" w418 {
        tunnel: w430 -> [_ w461]
        tunnel: [0 w459] -> w429
        frame False {
        }
        frame True {
          n172 = Add(x=w461, y=1) -> (x+y=w459:i32)
        }
      }
      n173 = feedback-in #10(w429) -> ()
      n174 = Greater?(x=w430, y=w424) -> (0:w425:bool)
      n175 = Greater?(x=w428, y=w424) -> (0:w426:bool)
      n176 = Greater?(x=w436, y=0.0) -> (0:w411:bool)
      n177 = Greater?(x=0.0, y=w436) -> (0:w416:bool)
      n178 = case shown="False" w407 {
        tunnel: w430 -> [_ _]
        tunnel: w425 -> [w465 _]
        tunnel: w426 -> [w464 w474]
        tunnel: [w463 w473] -> w406
        tunnel: w411 -> [w462 w472]
        frame False {
          n179 = case shown="False" w465 {
            tunnel: [w467 w471] -> w463
            tunnel: w464 -> [w468 _]
            tunnel: w462 -> [w466 _]
            frame False {
              n180 = case shown="False" w468 {
                tunnel: [w469 w470] -> w467
                tunnel: w466 -> [_ _]
                frame False {
                  w469 = T1 4 items=["Unknow", "Stable", "Following Warm", "Following Cold", "Unfollowing"]
                }
                frame True {
                  w470 = T1 4 items=["Unknow", "Stable", "Following Warm", "Following Cold", "Unfollowing"]
                }
              }
            }
            frame True {
              w471 = T1 1 items=["Unknow", "Stable", "Following Warm", "Following Cold", "Unfollowing"]
            }
          }
        }
        frame True {
          n181 = case shown="False" w474 {
            tunnel: [w475 w476] -> w473
            tunnel: w472 -> [_ w477]
            frame False {
              w475 = T1 4 items=["Unknow", "Stable", "Following Warm", "Following Cold", "Unfollowing"]
            }
            frame True {
              n182 = case shown="True" w477 {
                tunnel: [w478 w479] -> w476
                frame False {
                  w478 = T1 3 items=["Unknow", "Stable", "Following Warm", "Following Cold", "Unfollowing"]
                }
                frame True {
                  w479 = T1 2 items=["Unknow", "Stable", "Following Warm", "Following Cold", "Unfollowing"]
                }
              }
            }
          }
        }
      }
      "下拉列表" <- w406
      n183 = feedback #11() -> (w413:i32)  [unwired: 1 in]
      n184 = case shown="False" w411 {
        tunnel: [0 w440] -> w412
        tunnel: w413 -> [_ w442]
        tunnel: w410 -> [_ w441]
        tunnel: [FALSE w439] -> _
        frame False {
        }
        frame True {
          n185 = Add(x=w442, y=1) -> (x+y=w440:i32)
          n186 = Greater?(x=w440, y=w441) -> (0:w439:bool)
        }
      }
      n187 = feedback-in #11(w412) -> ()
      n188 = feedback #12() -> (w414:i32)  [unwired: 1 in]
      n189 = case shown="False" w416 {
        tunnel: [0 w448] -> w415
        tunnel: w414 -> [_ w449]
        tunnel: w410 -> [_ w447]
        tunnel: [FALSE w446] -> _
        frame False {
        }
        frame True {
          n190 = Add(x=w449, y=1) -> (x+y=w448:i32)
          n191 = Greater?(x=w448, y=w447) -> (0:w446:bool)
        }
      }
      n192 = feedback-in #12(w415) -> ()
    }
  }
  n193 = Bundle("Sensor Data"=w30, "Setpoint Value"=w29, "Heater Range"=w20, "Heater Output Value"=w28, "Ramp Active"=w25, w23, "Kelvin Reading"=w27, "Setpoint"=w17, "Heater Range"=w19, "Heater Output"=w26, "Ramping Active/Inactive"=w18, w16, FALSE) -> (→"output cluster":T2)  [unwired: 1 in]
